vi "Draw Line - Octant 0.vi"(5 "Delta y":i32, 6 "Colour":u32(colorbox), 7 "Delta x":i32, 8 "x Direction":i32, 9 "Y0":i32, 10 "X0":i32, 11 "Pixel Data in":u32[][](array[numeric])) -> (3 "Pixel Data out":u32[][](array[numeric]))   [LabVIEW 2022 SP3, in "Raster.lvlib"]
uses:
  Raster.lvlib
  <vilib>/Utility/High Resolution Relative Seconds.vi
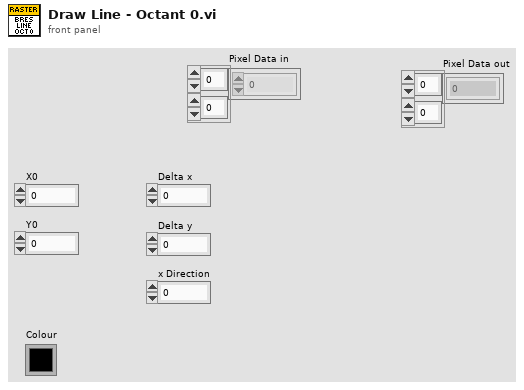
[diagram p1: front panel]
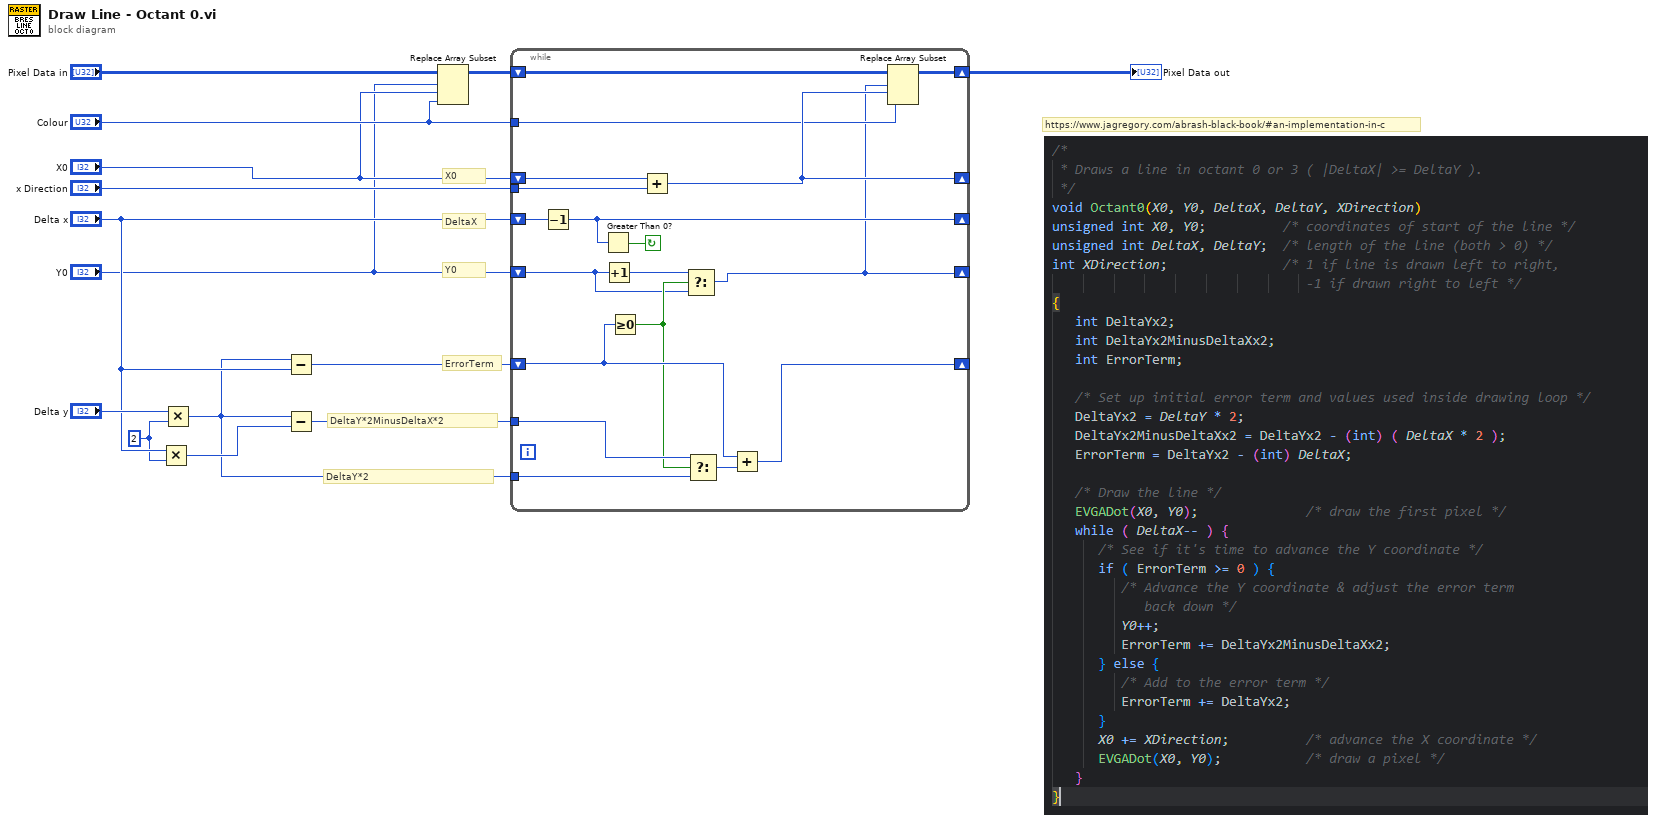
[diagram p0: block diagram]
diagram:
  w5 = 2 ("y")
  # "DeltaY*2"
  # "DeltaY*2MinusDeltaX*2"
  # "Y0"
  # "X0"
  # "DeltaX"
  # "https://www.jagregory.com/abrash-black-book/#an-implementation-in-c"
  # "ErrorTerm"
  n1 = Multiply(x="Delta x", y=w5) -> (x*y=w13:i32)
  n2 = Multiply(x="Delta y", y=w5) -> (x*y=w8:i32)
  n3 = Subtract(x=w8, y="Delta x") -> (x-y=w11:i32)
  n4 = Subtract(x=w8, y=w13) -> (x-y=w9:i32)
  n5 = Replace Array Subset(array="Pixel Data in", new element="Colour", index (row)="Y0", index (col)="X0") -> (w12:u32[][])
  n6 = while {
    shift-right: [w28] -> w1
    shift-left: w12 -> [w29]
    shift-right: [w30] -> _
    shift-left: w11 -> [w21]
    shift-right: [w23] -> _
    shift-left: "Delta x" -> [w32]
    shift-right: [w25] -> _
    shift-left: "X0" -> [w27]
    shift-right: [w16] -> _
    shift-left: "Y0" -> [w15]
    tunnel: w9 -> [w22]
    tunnel: w8 -> [w19]
    tunnel: "x Direction" -> [w26]
    tunnel: "Colour" -> [w24]
    stop <- w31 continue-if-true
    n7 = Decrement(x=w32) -> (x-1=w23:i32)
    n8 = Greater Than 0?(x=w23) -> (x > 0?=w31:bool)
    n9 = Increment(x=w15) -> (x+1=w17:i32)
    n10 = Greater Or Equal To 0?(x=w21) -> (x >= 0?=w18:bool)
    n11 = Add(x=w27, y=w26) -> (x+y=w25:i32)
    n12 = Select(t=w17, s=w18, f=w15) -> (s? t:f=w16:i32)
    n13 = Select(t=w22, s=w18, f=w19) -> (s? t:f=w20:i32)
    n14 = Add(x=w21, y=w20) -> (x+y=w30:i32)
    n15 = Replace Array Subset(array=w29, new element=w24, index (row)=w16, index (col)=w25) -> (w28:u32[][])
  }
  "Pixel Data out" <- w1
